vi "fw-fly-ctrl-init.vi"(11 "Linearsystem":T1) -> (0 "Kalman Error":errorcluster, 1 "LQR Error":bool, 2 "LinearQuadraticRegulator":T3, 3 "KalmanFilter":T4, 4 "Lin Sys Loop Error":bool, 5 "Linear System Loop":T5)   [LabVIEW 2019]
uses:
  <vilib>/Rock Robotics/WPI/ThirdParty/JAS_Junk/TrajLib/Trajectory_Library.lvlib
  <vilib>/Analysis/Matrix/Datatypes/RealMatrix.ctl
  <vilib>/Analysis/Matrix/NI_Matrix.lvlib
  <vilib>/Rock Robotics/WPI/ThirdParty/JAS_Junk/TrajLib/TypeDef/LINEAR_QUADRATIC_REGULATOR.ctl
  <vilib>/Rock Robotics/WPI/ThirdParty/JAS_Junk/TrajLib/TypeDef/LINEAR_PLANT_INV_FF.ctl
  <vilib>/Rock Robotics/WPI/ThirdParty/JAS_Junk/TrajLib/TypeDef/LINEAR_SYSTEM.ctl
  <vilib>/Rock Robotics/WPI/ThirdParty/JAS_Junk/TrajLib/TypeDef/KALMAN_FILTER.ctl
  <vilib>/Rock Robotics/WPI/ThirdParty/JAS_Junk/TrajLib/TypeDef/LINEAR_SYSTEM_LOOP.ctl
panel:
  # "<States,States>"
  # "<States,Inputs>"
  # "<Outputs,States>"
  # "<Outputs,Inputs>"
  # "Ref State <States,1>"
  # "Comp and capped \noutput <Inputs,1>"
  # "Controller gain\n<Inputs,States>"
  # "Steady State Gain  \n<States,Outputs>"
  # "State Estimate <Statess,1>"
  # "<States,States>"
  # "<States,Inputs>"
  # "<Outputs,States>"
  # "<Outputs,Inputs>"
  # "<States,1>"
  # "<FUTURE --- CLAMP TYPE -- For now\nuse Normalize>"
  # "Steady State Gain  \n<States,Outputs>"
  # "State Estimate <Statess,1>"
  # "<States,States>"
  # "<States,Inputs>"
  # "<Outputs,States>"
  # "<Outputs,Inputs>"
  # "<States,1>"
  # "<Inputs,1>"
  # "<States,Inputs>"
  # "<States,States>"
  # "Ref State <States,1>"
  # "Comp and capped \noutput <Inputs,1>"
  # "Controller gain\n<Inputs,States>"
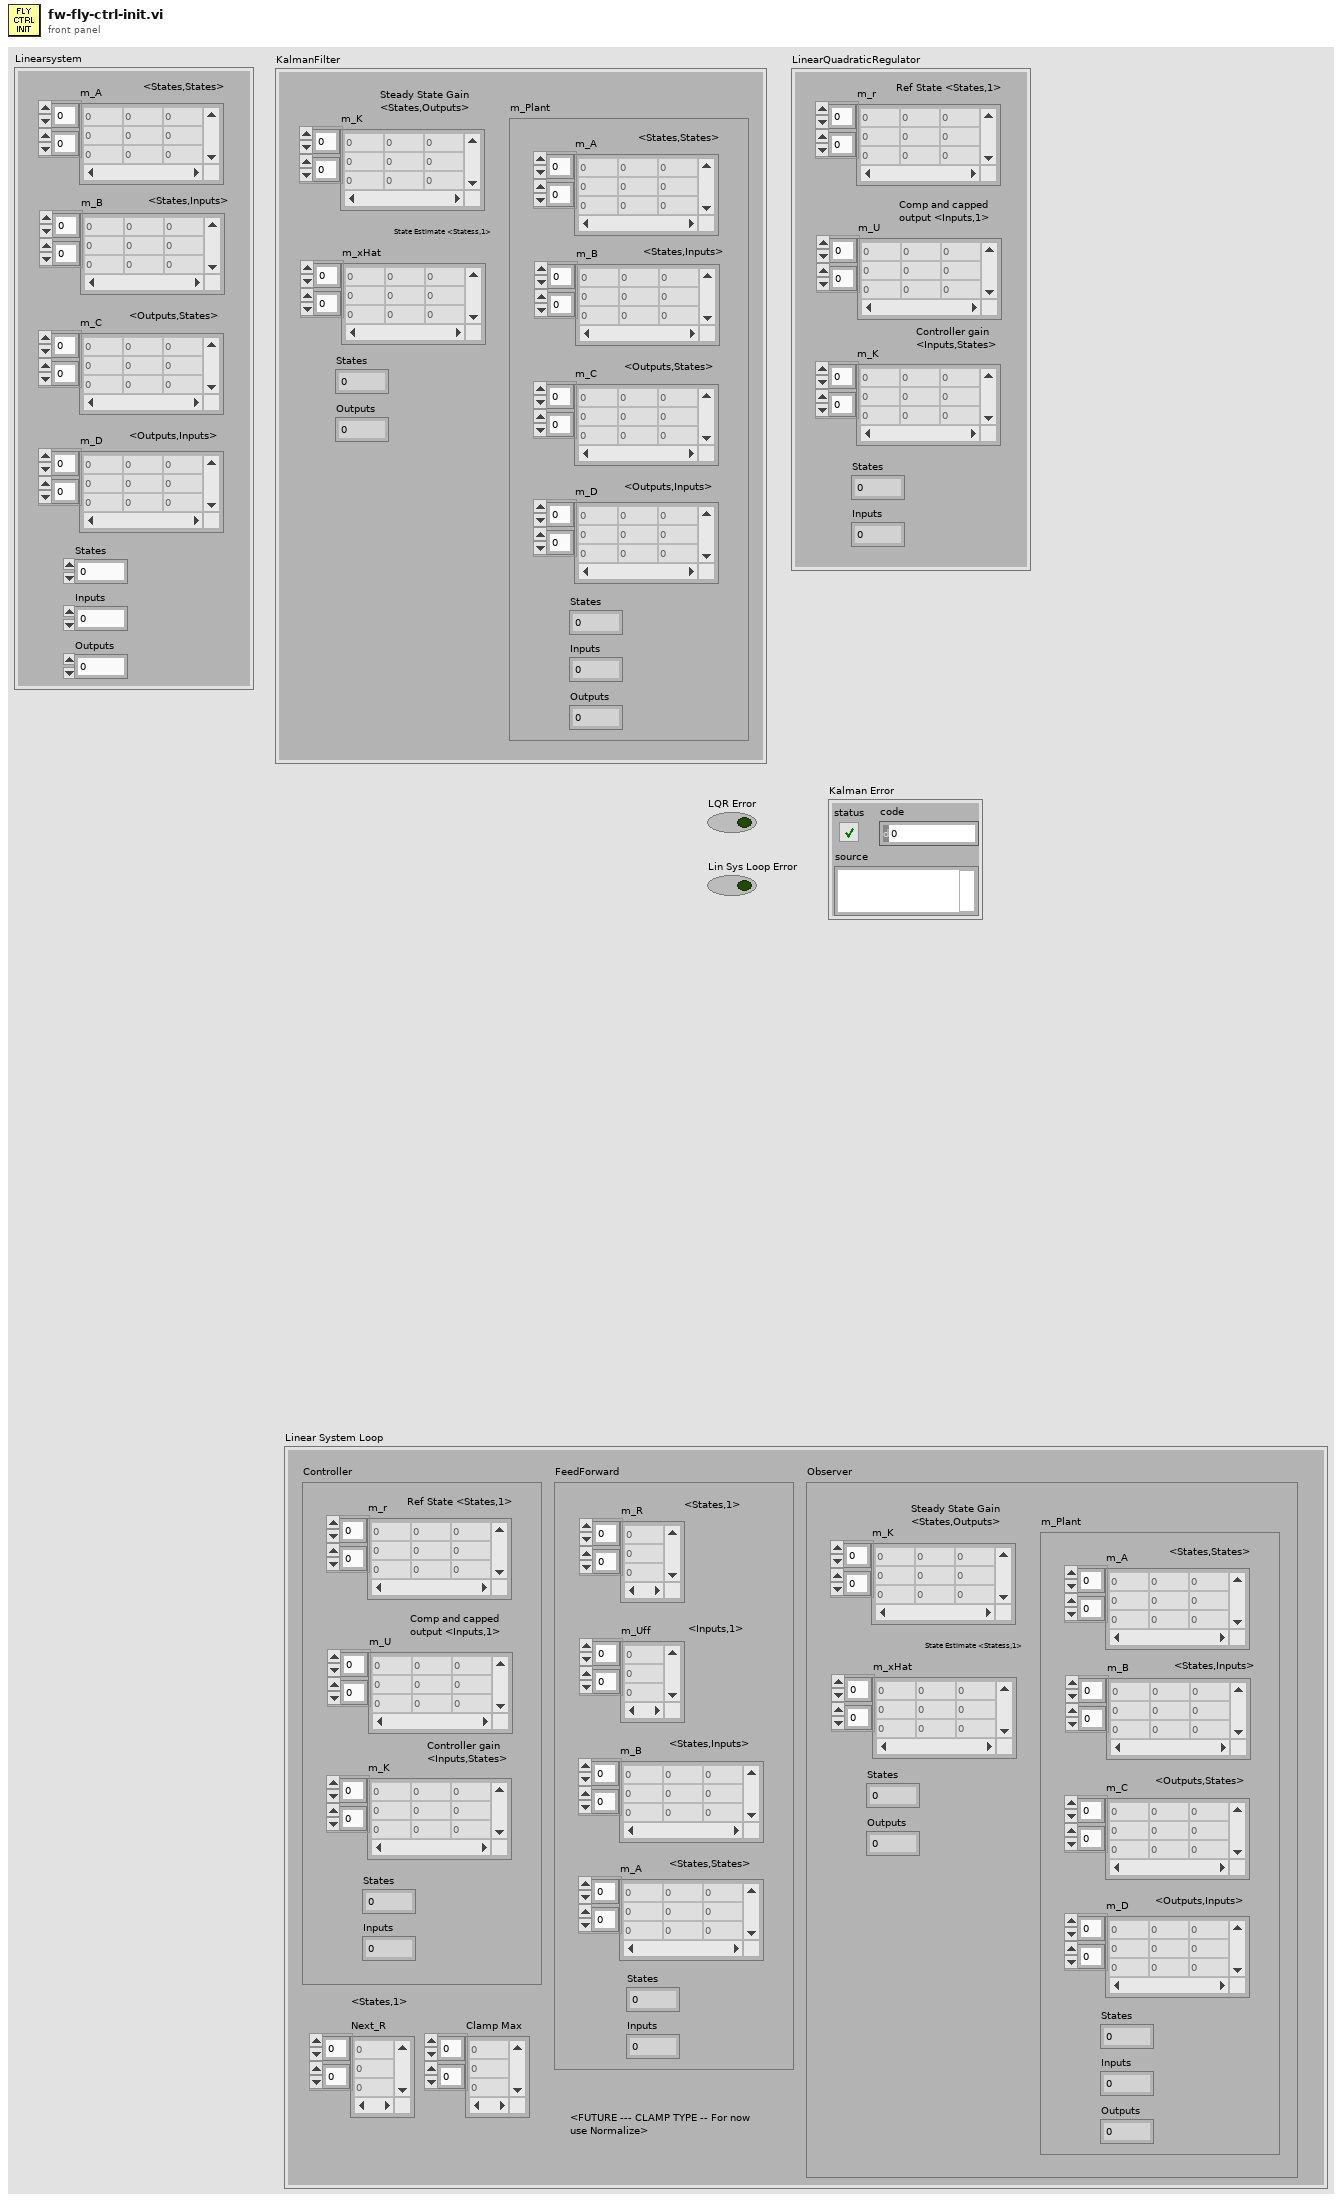
[diagram p1: front panel]
types:
  T1 = typedef "Trajectory_Library.lvlib/LINEAR_SYSTEM.ctl" = cluster{"m_A":T2, "m_B":T2, "m_C":T2, "m_D":T2, "States":i32, "Inputs":i32, "Outputs":i32}
  T2 = typedef "NI_Matrix.lvlib/RealMatrix.ctl" = dbl[][]
  T3 = typedef "Trajectory_Library.lvlib/LINEAR_QUADRATIC_REGULATOR.ctl" = cluster{"m_r":T2, "m_U":T2, "m_K":T2, "States":i32, "Inputs":i32}
  T4 = typedef "Trajectory_Library.lvlib/KALMAN_FILTER.ctl" = cluster{"m_K":T2, "m_xHat":T2, "States":i32, "Outputs":i32, "m_Plant":T1}
  T5 = typedef "Trajectory_Library.lvlib/LINEAR_SYSTEM_LOOP.ctl" = cluster{"Controller":T3, "FeedForward":T6, "Observer":T4, "Next_R":T2, "Clamp Max":T2}
  T6 = typedef "Trajectory_Library.lvlib/LINEAR_PLANT_INV_FF.ctl" = cluster{"m_R":T2, "m_Uff":T2, "m_B":T2, "m_A":T2, "States":i32, "Inputs":i32}
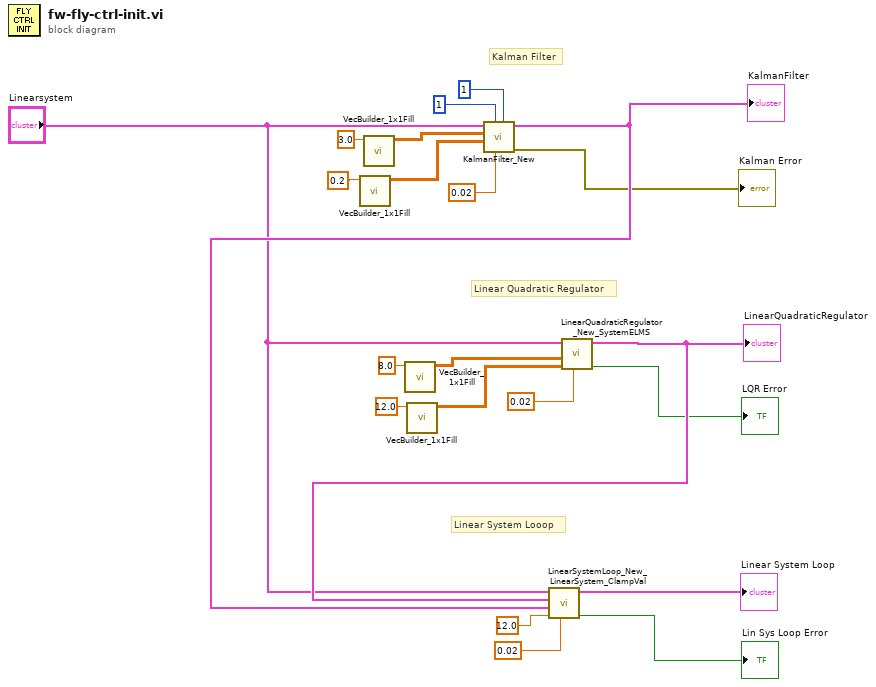
[diagram p0: block diagram]
diagram:
  # "Linear System Looop"
  # "Linear Quadratic Regulator"
  # "Kalman Filter"
  n1 = call <vilib>:"VecBuilder_1x1Fill.vi"("R0_C0"=0.2) -> ("output matrix"=w13:T2)  [unwired: 10 in]
  n2 = call <vilib>:"VecBuilder_1x1Fill.vi"("R0_C0"=3.0) -> ("output matrix"=w12:T2)  [unwired: 10 in]
  n3 = call <vilib>:"VecBuilder_1x1Fill.vi"("R0_C0"=8.0) -> ("output matrix"=w4:T2)  [unwired: 10 in]
  n4 = call <vilib>:"VecBuilder_1x1Fill.vi"("R0_C0"=12.0) -> ("output matrix"=w6:T2)  [unwired: 10 in]
  n5 = call <vilib>:"KalmanFilter_New.vi"("States"=1, "dt_Seconds"=0.02, "Outputs"=1, "MeasurementStdDevs"=w13, "StateStdDevs"=w12, "Plant"="Linearsystem") -> ("Error"=→"Kalman Error":errorcluster, "KalmanFilter"=w17:T4)  [unwired: 4 in]
  "KalmanFilter" <- w17
  n6 = call <vilib>:"LinearQuadraticRegulator_New_SystemELMS.vi"("dt_Seconds"=0.02, "Relms"=w6, "Qelms"=w4, "LINEARSYSTEM"="Linearsystem") -> ("Error"=→"LQR Error":bool, "LinearQuadraticRegulator"=w16:T3)  [unwired: 6 in]
  "LinearQuadraticRegulator" <- w16
  n7 = call <vilib>:"LinearSystemLoop_New_LinearSystem_ClampVal.vi"("dT_Seconds"=0.02, "Max_Voltage"=12.0, "Observer"=w17, "Controller"=w16, "Plant"="Linearsystem") -> ("Error"=→"Lin Sys Loop Error":bool, "Linear System Loop"=→"Linear System Loop":T5)  [unwired: 5 in]
